vi "Nand.vi"(2 "B":bool, 3 "A":bool) -> (0 "Output":bool)   [LabVIEW 2020, in "Hack.lvlib"]
uses:
  Hack.lvlib
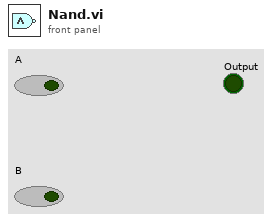
[diagram p1: front panel]
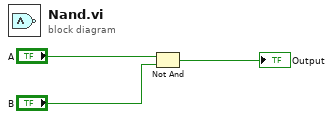
[diagram p0: block diagram]
diagram:
  n1 = Not And(1:"B", 2:"A") -> (0:→"Output":bool)
